vi "Generate Signal.vi"(8 "error in (no error)":errorcluster, 9 "Amplitude (1)":dbl=1.0, 10 "Frequency (1000 Hz)":dbl=1000.0, 11 "Signal Generation In":refnum<class "Signal Generation.lvclass">) -> (0 "error out":errorcluster, 3 "Signal Generation Out":refnum<class "Signal Generation.lvclass">)   [LabVIEW 2019, in "Signal Generation.lvclass"]
uses:
  Signal Generation.lvclass
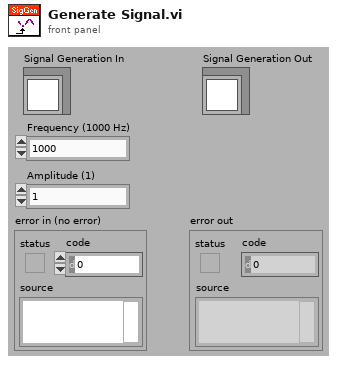
[diagram p1: front panel]
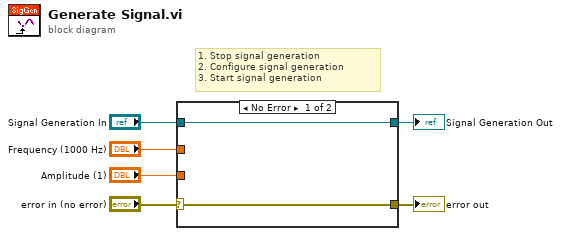
[diagram p0: block diagram]
diagram:
  # "1. Stop signal generation\n2. Configure signal generation\n3. Start signal generation"
  n1 = case shown="No Error" "error in (no error)" {
    selector: "error in (no error)" -> [w7 w10]
    tunnel: [w7 w10] -> w5
    tunnel: [w8 w9] -> w1
    tunnel: "Signal Generation In" -> [w8 w9]
    tunnel: "Frequency (1000 Hz)" -> [_ _]
    tunnel: "Amplitude (1)" -> [_ _]
    frame No Error {
    }
    frame Error {
    }
  }
  "error out" <- w5
  "Signal Generation Out" <- w1
